vi "Streaming.vi"(9 "Image Display Refnum":refnum<vi>, 10 "OnOff Refnum":refnum<vi>, 11 "camera":u64) -> ()   [LabVIEW 2019]
uses:
  EmergentCameraC/EmergentCameraC.lvlib
panel:
  in  "dshould":i32
  in  "dusing":i32
  in  "frame2":T1
  in  "frame1":T1
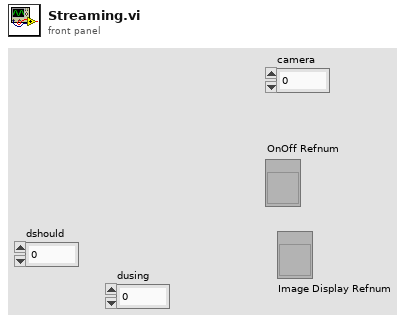
[diagram p1: front panel]
types:
  T1 = cluster{"pixel_type":u32, "size_x":u32, "size_y":u32, "stride":i32, "offset_x":u32, "offset_y":u32, "padding_x":u32, "padding_y":u32, "trailer_size_y":u32, "frame_id":u16, "@dummy control@":i8, "@dummy control@":i8, "imagePtr":i64, "bufferSize":u32, "@dummy control@":i8, "@dummy control@":i8, "@dummy control@":i8, "@dummy control@":i8, "timestamp":u64, "nsecs":u64, "convertColor":i32, "convertBitDepth":i32, "privateData[0]":u8, "privateData[1]":u8, "privateData[2]":u8, "privateData[3]":u8, "privateData[4]":u8, "privateData[5]":u8, "privateData[6]":u8, "privateData[7]":u8, "privateData[8]":u8, "privateData[9]":u8, "privateData[10]":u8, "privateData[11]":u8, "privateData[12]":u8, "privateData[13]":u8, "privateData[14]":u8, "privateData[15]":u8, "privateData[16]":u8, "privateData[17]":u8, "privateData[18]":u8, "privateData[19]":u8, "privateData[20]":u8, "privateData[21]":u8, "privateData[22]":u8, "privateData[23]":u8, "privateData[24]":u8, "privateData[25]":u8, "privateData[26]":u8, "privateData[27]":u8, "privateData[28]":u8, "privateData[29]":u8, "privateData[30]":u8, "privateData[31]":u8, "privateData[32]":u8, "privateData[33]":u8, "privateData[34]":u8, "privateData[35]":u8, "privateData[36]":u8, "privateData[37]":u8, "privateData[38]":u8, "privateData[39]":u8, "privateData[40]":u8, "privateData[41]":u8, "privateData[42]":u8, "privateData[43]":u8, "privateData[44]":u8, "privateData[45]":u8, "privateData[46]":u8, "privateData[47]":u8, "privateData[48]":u8, "privateData[49]":u8, "privateData[50]":u8, "privateData[51]":u8, "privateData[52]":u8, "privateData[53]":u8, "privateData[54]":u8, "privateData[55]":u8, "privateData[56]":u8, "privateData[57]":u8, "privateData[58]":u8, "privateData[59]":u8, "privateData[60]":u8, "privateData[61]":u8, "privateData[62]":u8, "privateData[63]":u8, "privateData[64]":u8, "privateData[65]":u8, "privateData[66]":u8, "privateData[67]":u8, "privateData[68]":u8, "privateData[69]":u8, "privateData[70]":u8, "privateData[71]":u8, "privateData[72]":u8, "privateData[73]":u8, "privateData[74]":u8, "privateData[75]":u8, "privateData[76]":u8, "privateData[77]":u8, "privateData[78]":u8, "privateData[79]":u8, "privateData[80]":u8, "privateData[81]":u8, "privateData[82]":u8, "privateData[83]":u8, "privateData[84]":u8, "privateData[85]":u8, "privateData[86]":u8, "privateData[87]":u8, "privateData[88]":u8, "privateData[89]":u8, "privateData[90]":u8, "privateData[91]":u8, "privateData[92]":u8, "privateData[93]":u8, "privateData[94]":u8, "privateData[95]":u8, "privateData[96]":u8, "privateData[97]":u8, "privateData[98]":u8, "privateData[99]":u8, "privateData[100]":u8, "privateData[101]":u8, "privateData[102]":u8, "privateData[103]":u8, "privateData[104]":u8, "privateData[105]":u8, "privateData[106]":u8, "privateData[107]":u8, "privateData[108]":u8, "privateData[109]":u8, "privateData[110]":u8, "privateData[111]":u8, "privateData[112]":u8, "privateData[113]":u8, "privateData[114]":u8, "privateData[115]":u8, "privateData[116]":u8, "privateData[117]":u8, "privateData[118]":u8, "privateData[119]":u8, "privateData[120]":u8, "privateData[121]":u8, "privateData[122]":u8, "privateData[123]":u8, "privateData[124]":u8, "privateData[125]":u8, "privateData[126]":u8, "privateData[127]":u8, "privateData[128]":u8, "privateData[129]":u8, "privateData[130]":u8, "privateData[131]":u8, "privateData[132]":u8, "privateData[133]":u8, "privateData[134]":u8, "privateData[135]":u8, "privateData[136]":u8, "privateData[137]":u8, "privateData[138]":u8, "privateData[139]":u8, "privateData[140]":u8, "privateData[141]":u8, "privateData[142]":u8, "privateData[143]":u8, "privateData[144]":u8, "privateData[145]":u8, "privateData[146]":u8, "privateData[147]":u8, "privateData[148]":u8, "privateData[149]":u8, "privateData[150]":u8, "privateData[151]":u8, "privateData[152]":u8, "privateData[153]":u8, "privateData[154]":u8, "privateData[155]":u8, "privateData[156]":u8, "privateData[157]":u8, "privateData[158]":u8, "privateData[159]":u8, "privateData[160]":u8, "privateData[161]":u8, "privateData[162]":u8, "privateData[163]":u8, "privateData[164]":u8, "privateData[165]":u8, "privateData[166]":u8, "privateData[167]":u8, "privateData[168]":u8, "privateData[169]":u8, "privateData[170]":u8, "privateData[171]":u8, "privateData[172]":u8, "privateData[173]":u8, "privateData[174]":u8, "privateData[175]":u8, "privateData[176]":u8, "privateData[177]":u8, "privateData[178]":u8, "privateData[179]":u8, "privateData[180]":u8, "privateData[181]":u8, "privateData[182]":u8, "privateData[183]":u8, "privateData[184]":u8, "privateData[185]":u8, "privateData[186]":u8, "privateData[187]":u8, "privateData[188]":u8, "privateData[189]":u8, "privateData[190]":u8, "privateData[191]":u8, "privateData[192]":u8, "privateData[193]":u8, "privateData[194]":u8, "privateData[195]":u8, "privateData[196]":u8, "privateData[197]":u8, "privateData[198]":u8, "privateData[199]":u8, "privateData[200]":u8, "privateData[201]":u8, "privateData[202]":u8, "privateData[203]":u8, "privateData[204]":u8, "privateData[205]":u8, "privateData[206]":u8, "privateData[207]":u8, "privateData[208]":u8, "privateData[209]":u8, "privateData[210]":u8, "privateData[211]":u8, "privateData[212]":u8, "privateData[213]":u8, "privateData[214]":u8, "privateData[215]":u8, "privateData[216]":u8, "privateData[217]":u8, "privateData[218]":u8, "privateData[219]":u8, "privateData[220]":u8, "privateData[221]":u8, "privateData[222]":u8, "privateData[223]":u8, "privateData[224]":u8, "privateData[225]":u8, "privateData[226]":u8, "privateData[227]":u8, "privateData[228]":u8, "privateData[229]":u8, "privateData[230]":u8, "privateData[231]":u8, "privateData[232]":u8, "privateData[233]":u8, "privateData[234]":u8, "privateData[235]":u8, "privateData[236]":u8, "privateData[237]":u8, "privateData[238]":u8, "privateData[239]":u8, "privateData[240]":u8, "privateData[241]":u8, "privateData[242]":u8, "privateData[243]":u8, "privateData[244]":u8, "privateData[245]":u8, "privateData[246]":u8, "privateData[247]":u8, "privateData[248]":u8, "privateData[249]":u8, "privateData[250]":u8, "privateData[251]":u8, "privateData[252]":u8, "privateData[253]":u8, "privateData[254]":u8, "privateData[255]":u8}
  T2 = cluster{"pixel_type":u32, "size_x":u32, "size_y":u32, "stride":i32, "offset_x":u32, "offset_y":u32, "padding_x":u32, "padding_y":u32, "trailer_size_y":u32, "frame_id":u16, "@dummy control@":i8, "@dummy control@":i8, "imagePtr":i64, "bufferSize":u32, "@dummy control@":i8, "@dummy control@":i8, "@dummy control@":i8, "@dummy control@":i8, "timestamp":u64, "nsecs":u64, "convertColor":i32, "convertBitDepth":i32, "privateData[0]":u8, "privateData[1]":u8, "privateData[2]":u8, "privateData[3]":u8, "privateData[4]":u8, "privateData[5]":u8, "privateData[6]":u8, "privateData[7]":u8, "privateData[8]":u8, "privateData[9]":u8, "privateData[10]":u8, "privateData[11]":u8, "privateData[12]":u8, "privateData[13]":u8, "privateData[14]":u8, "privateData[15]":u8, "privateData[16]":u8, "privateData[17]":u8, "privateData[18]":u8, "privateData[19]":u8, "privateData[20]":u8, "privateData[21]":u8, "privateData[22]":u8, "privateData[23]":u8, "privateData[24]":u8, "privateData[25]":u8, "privateData[26]":u8, "privateData[27]":u8, "privateData[28]":u8, "privateData[29]":u8, "privateData[30]":u8, "privateData[31]":u8, "privateData[32]":u8, "privateData[33]":u8, "privateData[34]":u8, "privateData[35]":u8, "privateData[36]":u8, "privateData[37]":u8, "privateData[38]":u8, "privateData[39]":u8, "privateData[40]":u8, "privateData[41]":u8, "privateData[42]":u8, "privateData[43]":u8, "privateData[44]":u8, "privateData[45]":u8, "privateData[46]":u8, "privateData[47]":u8, "privateData[48]":u8, "privateData[49]":u8, "privateData[50]":u8, "privateData[51]":u8, "privateData[52]":u8, "privateData[53]":u8, "privateData[54]":u8, "privateData[55]":u8, "privateData[56]":u8, "privateData[57]":u8, "privateData[58]":u8, "privateData[59]":u8, "privateData[60]":u8, "privateData[61]":u8, "privateData[62]":u8, "privateData[63]":u8, "privateData[64]":u8, "privateData[65]":u8, "privateData[66]":u8, "privateData[67]":u8, "privateData[68]":u8, "privateData[69]":u8, "privateData[70]":u8, "privateData[71]":u8, "privateData[72]":u8, "privateData[73]":u8, "privateData[74]":u8, "privateData[75]":u8, "privateData[76]":u8, "privateData[77]":u8, "privateData[78]":u8, "privateData[79]":u8, "privateData[80]":u8, "privateData[81]":u8, "privateData[82]":u8, "privateData[83]":u8, "privateData[84]":u8, "privateData[85]":u8, "privateData[86]":u8, "privateData[87]":u8, "privateData[88]":u8, "privateData[89]":u8, "privateData[90]":u8, "privateData[91]":u8, "privateData[92]":u8, "privateData[93]":u8, "privateData[94]":u8, "privateData[95]":u8, "privateData[96]":u8, "privateData[97]":u8, "privateData[98]":u8, "privateData[99]":u8, "privateData[100]":u8, "privateData[101]":u8, "privateData[102]":u8, "privateData[103]":u8, "privateData[104]":u8, "privateData[105]":u8, "privateData[106]":u8, "privateData[107]":u8, "privateData[108]":u8, "privateData[109]":u8, "privateData[110]":u8, "privateData[111]":u8, "privateData[112]":u8, "privateData[113]":u8, "privateData[114]":u8, "privateData[115]":u8, "privateData[116]":u8, "privateData[117]":u8, "privateData[118]":u8, "privateData[119]":u8, "privateData[120]":u8, "privateData[121]":u8, "privateData[122]":u8, "privateData[123]":u8, "privateData[124]":u8, "privateData[125]":u8, "privateData[126]":u8, "privateData[127]":u8, "privateData[128]":u8, "privateData[129]":u8, "privateData[130]":u8, "privateData[131]":u8, "privateData[132]":u8, "privateData[133]":u8, "privateData[134]":u8, "privateData[135]":u8, "privateData[136]":u8, "privateData[137]":u8, "privateData[138]":u8, "privateData[139]":u8, "privateData[140]":u8, "privateData[141]":u8, "privateData[142]":u8, "privateData[143]":u8, "privateData[144]":u8, "privateData[145]":u8, "privateData[146]":u8, "privateData[147]":u8, "privateData[148]":u8, "privateData[149]":u8, "privateData[150]":u8, "privateData[151]":u8, "privateData[152]":u8, "privateData[153]":u8, "privateData[154]":u8, "privateData[155]":u8, "privateData[156]":u8, "privateData[157]":u8, "privateData[158]":u8, "privateData[159]":u8, "privateData[160]":u8, "privateData[161]":u8, "privateData[162]":u8, "privateData[163]":u8, "privateData[164]":u8, "privateData[165]":u8, "privateData[166]":u8, "privateData[167]":u8, "privateData[168]":u8, "privateData[169]":u8, "privateData[170]":u8, "privateData[171]":u8, "privateData[172]":u8, "privateData[173]":u8, "privateData[174]":u8, "privateData[175]":u8, "privateData[176]":u8, "privateData[177]":u8, "privateData[178]":u8, "privateData[179]":u8, "privateData[180]":u8, "privateData[181]":u8, "privateData[182]":u8, "privateData[183]":u8, "privateData[184]":u8, "privateData[185]":u8, "privateData[186]":u8, "privateData[187]":u8, "privateData[188]":u8, "privateData[189]":u8, "privateData[190]":u8, "privateData[191]":u8, "privateData[192]":u8, "privateData[193]":u8, "privateData[194]":u8, "privateData[195]":u8, "privateData[196]":u8, "privateData[197]":u8, "privateData[198]":u8, "privateData[199]":u8, "privateData[200]":u8, "privateData[201]":u8, "privateData[202]":u8, "privateData[203]":u8, "privateData[204]":u8, "privateData[205]":u8, "privateData[206]":u8, "privateData[207]":u8, "privateData[208]":u8, "privateData[209]":u8, "privateData[210]":u8, "privateData[211]":u8, "privateData[212]":u8, "privateData[213]":u8, "privateData[214]":u8, "privateData[215]":u8, "privateData[216]":u8, "privateData[217]":u8, "privateData[218]":u8, "privateData[219]":u8, "privateData[220]":u8, "privateData[221]":u8, "privateData[222]":u8, "privateData[223]":u8, "privateData[224]":u8, "privateData[225]":u8, "privateData[226]":u8, "privateData[227]":u8, "privateData[228]":u8, "privateData[229]":u8, "privateData[230]":u8, "privateData[231]":u8, "privateData[232]":u8, "privateData[233]":u8, "privateData[234]":u8, "privateData[235]":u8, "privateData[236]":u8, "privateData[237]":u8, "privateData[238]":u8, "privateData[239]":u8, "privateData[240]":u8, "privateData[241]":u8, "privateData[242]":u8, "privateData[243]":u8, "privateData[244]":u8, "privateData[245]":u8, "privateData[246]":u8, "privateData[247]":u8, "privateData[248]":u8, "privateData[249]":u8, "privateData[250]":u8, "privateData[251]":u8, "privateData[252]":u8, "privateData[253]":u8, "privateData[254]":u8, "privateData[255]":u8}[]
  T3 = typedef "Image Type" = u32
  T4 = typedef "Semaphore RefNum" = refnum<k1>
  T5 = typedef "IMAQ Image.ctl" = refnum<image>
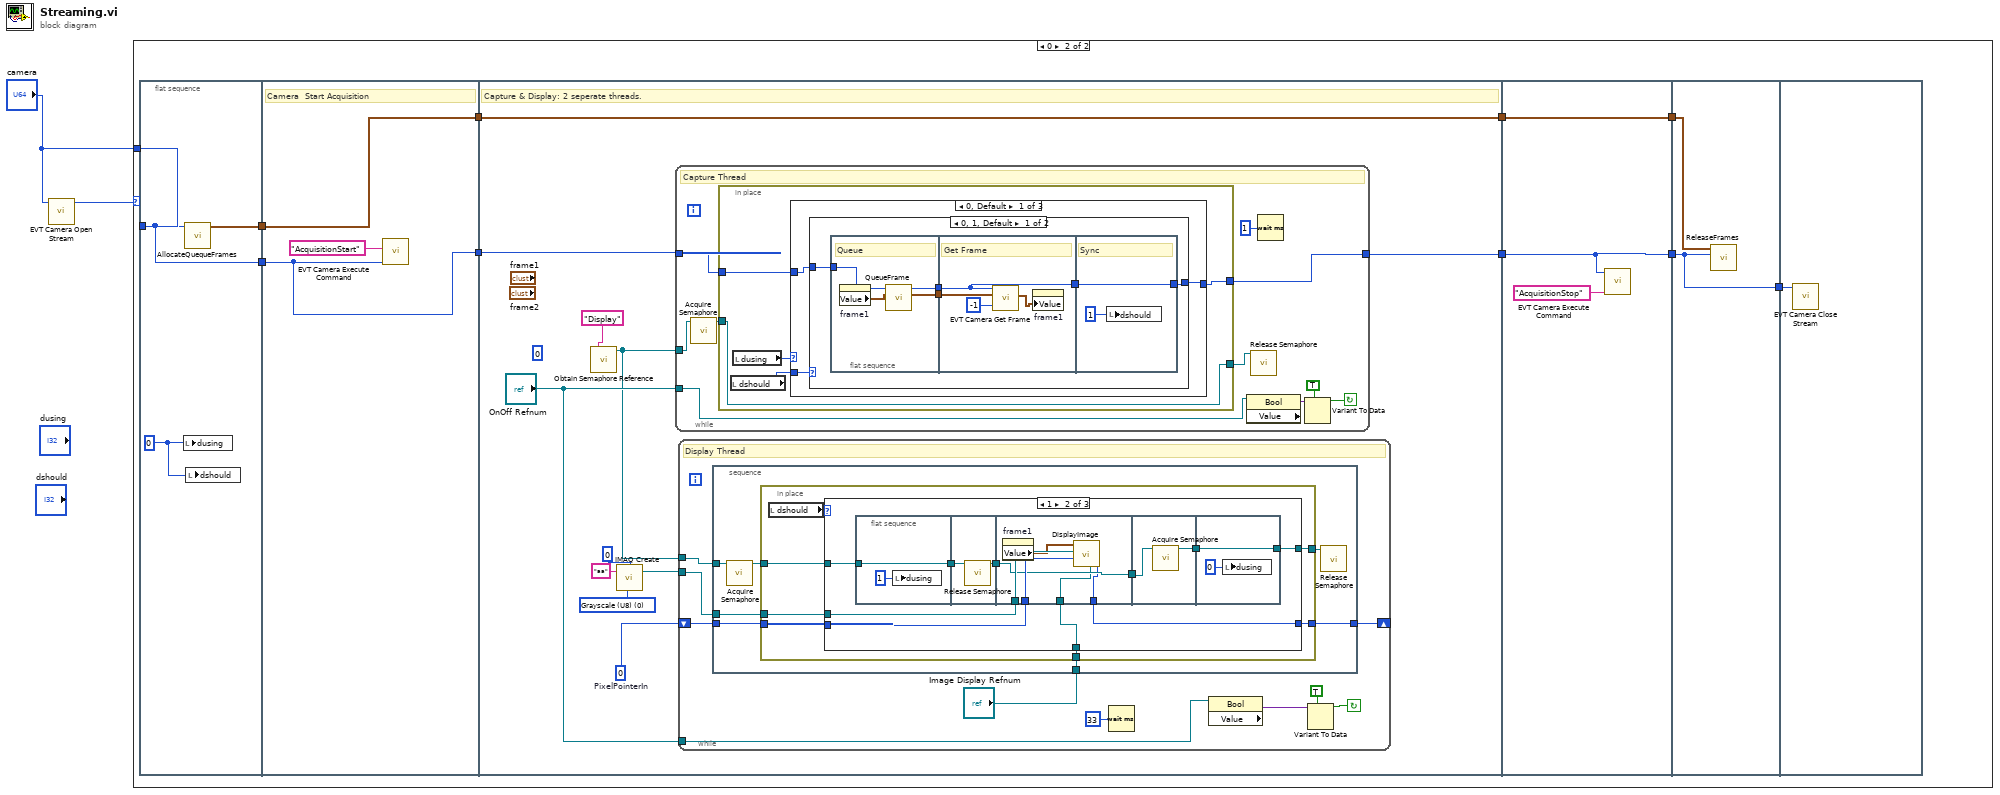
[diagram p0: block diagram]
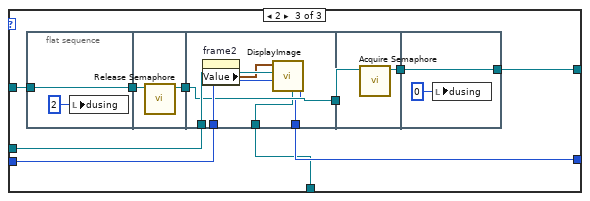
[diagram p4: hidden frame]
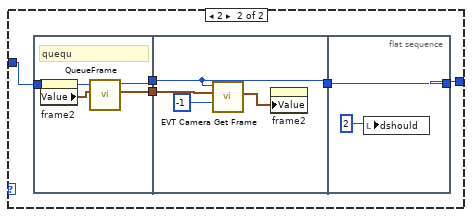
[diagram p5: hidden frame]
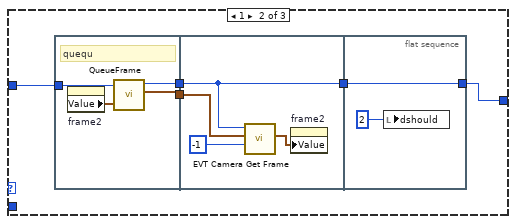
[diagram p6: hidden frame]
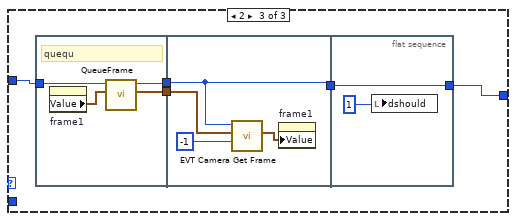
[diagram p7: hidden frame]
diagram:
  n1 = call "EVT Camera Open Stream.vi"("camera"="camera") -> ("function return"=w1:u32)  [unwired: 10 in]
  n2 = case shown="0" w1 {
    tunnel: "camera" -> [_ w3]
    frame Default {
    }
    frame 0 {
      n3 = flat-sequence {
        tunnel: [w15] -> w12
        tunnel: w3 -> [w14]
        tunnel: [w14] -> w11
        tunnel: w12 -> [w18]
        tunnel: w11 -> [w17]
        tunnel: [w18] -> w10
        tunnel: [w17] -> w4
        tunnel: w10 -> [w29]
        tunnel: [w28] -> w9
        tunnel: [w29] -> w8
        tunnel: w4 -> [w27]
        tunnel: w9 -> [w183]
        tunnel: w8 -> [w182]
        tunnel: [w183] -> w7
        tunnel: [w182] -> w6
        tunnel: w7 -> [w185]
        tunnel: w6 -> [w186]
        tunnel: [w185] -> w5
        tunnel: w5 -> [w187]
        frame #0 {
          w13 = 0 ("frameDisplayUse")
          n4 = local write "dusing"(w13) -> ()
          n5 = call "AllocateQuequeFrames.vi"("camera"=w14) -> ("Array"=w15:T2)  [unwired: 9 in, 1 out]
          n6 = local write "dshould"(w13) -> ()
        }
        frame #1 {
          # "Camera  Start Acquisition"
          n7 = call "EVT Camera Execute Command.vi"("name"="AcquisitionStart", "camera"=w17) -> ()  [unwired: 9 in, 1 out]
        }
        frame #2 {
          w19 = T3 0 items=["Grayscale (U8)", "Grayscale (I16)", "Grayscale (SGL)", "Complex (CSG)", "RGB (U32)", "HSL (U32)", "RGB (U64)", "Grayscale (U16)"] ("Image Type")
          w21 = u64 0  # PixelPointerIn
          (unwired) u16 0 ("op")
          # "Capture & Display: 2 seperate threads."
          n8 = call <vilib>:"Obtain Semaphore Reference.vi"("name (unnamed)"="Display") -> ("semaphore"=w24:T4)  [unwired: 4 in, 2 out]
          n9 = call "IMAQ Create"("Border Size"=0, "Image Name"="aa", "Image Type"=w19) -> ("New Image"=w20:T5)  [unwired: 2 in, 1 out]
          n10 = while "Capture thread" {
            tunnel: w27 -> [w108]
            tunnel: [w104] -> w28
            tunnel: w24 -> [w109]
            tunnel: "OnOff Refnum" -> [w105]
            stop <- w110 continue-if-true
            # "Capture Thread"
            n11 = call <vilib>:"Acquire Semaphore.vi"("semaphore"=w109) -> ("semaphore out"=w107:T4)  [unwired: 4 in, 2 out]
            n12 = in-place {
              in-place-border: w108 -> [w118]
              in-place-border: w107 -> [w115]
              in-place-border: [w115] -> w106
              in-place-border: [w114] -> w104
              n13 = local read "dshould"() -> (w116:i32)
              n14 = local read "dusing"() -> (w117:i32)
              n15 = case shown="0, Default" w117 {
                tunnel: w118 -> [w121 w154 w168]
                tunnel: [w120 w152 w167] -> w114
                tunnel: w116 -> [w119 _ _]
                frame 0, Default {
                  n16 = case shown="0, 1, Default" w119 {
                    tunnel: w121 -> [w124 w137]
                    tunnel: [w123 w138] -> w120
                    frame 0, 1, Default {
                      n17 = flat-sequence {
                        tunnel: w124 -> [w130]
                        tunnel: [w127] -> w126
                        tunnel: [w129] -> w122
                        tunnel: w126 -> [w133]
                        tunnel: [w132] -> w125
                        tunnel: w122 -> [w132]
                        tunnel: [w136] -> w123
                        tunnel: w125 -> [w136]
                        frame #0 {
                          # "Queue"
                          n18 = property on="frame1" class="Clust (strict)"() -> ("Value"=w128:T1)  [unwired: 2 in, 2 out]
                          n19 = call "QueueFrame.vi"("frame"=w128, "camera"=w130) -> ("frame_out"=w127:T1, "camera_out"=w129:u64)  [unwired: 8 in]
                        }
                        frame #1 {
                          # "Get Frame"
                          n20 = call "EVT Camera Get Frame.vi"("timeout"=-1, "frame"=w133, "camera"=w132) -> ("frame out"=w131:T1)  [unwired: 7 in, 1 out]
                          n21 = property on="frame1" class="Clust (strict)"("Value"=w131) -> ()  [unwired: 2 in, 2 out]
                        }
                        frame #2 {
                          # "Sync"
                          n22 = local write "dshould"(1 ("DisplayFrame")) -> ()
                        }
                      }
                    }
                    frame 2 {
                      n23 = flat-sequence {
                        tunnel: w137 -> [w145]
                        tunnel: [w143] -> w141
                        tunnel: [w144] -> w140
                        tunnel: w141 -> [w148]
                        tunnel: w140 -> [w147]
                        tunnel: [w147] -> w139
                        tunnel: [w150] -> w138
                        tunnel: w139 -> [w150]
                        frame #0 {
                          # "quequ"
                          n24 = property on="frame2" class="Clust (strict)"() -> ("Value"=w142:T1)  [unwired: 2 in, 2 out]
                          n25 = call "QueueFrame.vi"("frame"=w142, "camera"=w145) -> ("frame_out"=w143:T1, "camera_out"=w144:u64)  [unwired: 8 in]
                        }
                        frame #1 {
                          n26 = call "EVT Camera Get Frame.vi"("timeout"=-1, "frame"=w148, "camera"=w147) -> ("frame out"=w146:T1)  [unwired: 7 in, 1 out]
                          n27 = property on="frame2" class="Clust (strict)"("Value"=w146) -> ()  [unwired: 2 in, 2 out]
                        }
                        frame #2 {
                          n28 = local write "dshould"(2 ("DisplayFrame")) -> ()
                        }
                      }
                    }
                  }
                }
                frame 1 {
                  n29 = flat-sequence {
                    tunnel: w154 -> [w160]
                    tunnel: [w158] -> w156
                    tunnel: [w159] -> w155
                    tunnel: w156 -> [w163]
                    tunnel: w155 -> [w162]
                    tunnel: [w162] -> w153
                    tunnel: [w165] -> w152
                    tunnel: w153 -> [w165]
                    frame #0 {
                      # "quequ"
                      n30 = property on="frame2" class="Clust (strict)"() -> ("Value"=w157:T1)  [unwired: 2 in, 2 out]
                      n31 = call "QueueFrame.vi"("frame"=w157, "camera"=w160) -> ("frame_out"=w158:T1, "camera_out"=w159:u64)  [unwired: 8 in]
                    }
                    frame #1 {
                      n32 = call "EVT Camera Get Frame.vi"("timeout"=-1, "frame"=w163, "camera"=w162) -> ("frame out"=w161:T1)  [unwired: 7 in, 1 out]
                      n33 = property on="frame2" class="Clust (strict)"("Value"=w161) -> ()  [unwired: 2 in, 2 out]
                    }
                    frame #2 {
                      n34 = local write "dshould"(2 ("DisplayFrame")) -> ()
                    }
                  }
                }
                frame 2 {
                  n35 = flat-sequence {
                    tunnel: w168 -> [w175]
                    tunnel: [w173] -> w171
                    tunnel: [w174] -> w170
                    tunnel: w171 -> [w178]
                    tunnel: w170 -> [w177]
                    tunnel: [w177] -> w169
                    tunnel: [w181] -> w167
                    tunnel: w169 -> [w181]
                    frame #0 {
                      # "quequ"
                      n36 = property on="frame1" class="Clust (strict)"() -> ("Value"=w172:T1)  [unwired: 2 in, 2 out]
                      n37 = call "QueueFrame.vi"("frame"=w172, "camera"=w175) -> ("frame_out"=w173:T1, "camera_out"=w174:u64)  [unwired: 8 in]
                    }
                    frame #1 {
                      n38 = call "EVT Camera Get Frame.vi"("timeout"=-1, "frame"=w178, "camera"=w177) -> ("frame out"=w176:T1)  [unwired: 7 in, 1 out]
                      n39 = property on="frame1" class="Clust (strict)"("Value"=w176) -> ()  [unwired: 2 in, 2 out]
                    }
                    frame #2 {
                      n40 = local write "dshould"(1 ("DisplayFrame")) -> ()
                    }
                  }
                }
              }
            }
            n41 = property class="Bool"(reference=w105) -> ("Value"=w112:variant)  [unwired: 1 in, 2 out]
            n42 = call <vilib>:"Release Semaphore.vi"("semaphore"=w106) -> ()  [unwired: 5 in, 2 out]
            n43 = Wait (ms)(milliseconds to wait=u32 1) -> ()  [unwired: 1 out]
            n44 = Variant To Data(type=TRUE, Variant=w112) -> (data=w110:bool)  [unwired: 1 in, 1 out]
          }
          n45 = while {
            tunnel: w20 -> [w33]
            shift-right: [w32] -> _
            shift-left: w21 -> [w34]
            tunnel: w24 -> [w35]
            tunnel: "OnOff Refnum" -> [w30]
            stop <- w36 continue-if-true
            # "Display Thread"
            n46 = stacked-sequence {
              tunnel: w34 -> [w46]
              tunnel: w35 -> [w45]
              tunnel: w33 -> [w43]
              tunnel: [w42] -> w32
              tunnel: "Image Display Refnum" -> [w40]
              frame #0 {
                n47 = call <vilib>:"Acquire Semaphore.vi"("semaphore"=w45) -> ("semaphore out"=w44:T4)  [unwired: 4 in, 2 out]
                n48 = in-place {
                  in-place-border: w46 -> [w52]
                  in-place-border: w44 -> [w51]
                  in-place-border: w43 -> [w50]
                  in-place-border: [w49] -> w41
                  in-place-border: [w48] -> w42
                  in-place-border: w40 -> [w47]
                  n49 = local read "dshould"() -> (w53:i32)
                  n50 = case shown="1" w53 {
                    tunnel: w52 -> [w54 w62 w86]
                    tunnel: w51 -> [w55 w65 w89]
                    tunnel: w50 -> [_ w63 w87]
                    tunnel: [w55 w58 w82] -> w49
                    tunnel: [w54 w57 w81] -> w48
                    tunnel: w47 -> [_ w56 w80]
                    frame 0, Default {
                    }
                    frame 1 {
                      n51 = flat-sequence {
                        tunnel: w65 -> [w66]
                        tunnel: [w66] -> w64
                        tunnel: w64 -> [w69]
                        tunnel: [w68] -> w61
                        tunnel: w63 -> [w75]
                        tunnel: w62 -> [w74]
                        tunnel: w61 -> [w73]
                        tunnel: [w73] -> w60
                        tunnel: [w72] -> w57
                        tunnel: w56 -> [w71]
                        tunnel: w60 -> [w77]
                        tunnel: [w76] -> w59
                        tunnel: [w79] -> w58
                        tunnel: w59 -> [w79]
                        frame #0 {
                          n52 = local write "dusing"(1 ("dusing")) -> ()
                        }
                        frame #1 {
                          n53 = call <vilib>:"Release Semaphore.vi"("semaphore"=w69) -> ("semaphore out"=w68:T4)  [unwired: 5 in, 1 out]
                        }
                        frame #2 {
                          n54 = property on="frame1" class="Clust (strict)"() -> ("Value"=w70:T1)  [unwired: 2 in, 2 out]
                          n55 = call "DisplayImage.vi"("frame"=w70, "ImageIMAQ"=w75, "PixelPointerIn"=w74, "Image Display Refnum"=w71) -> ("PixelPointerOut"=w72:u64)  [unwired: 4 in, 1 out]
                        }
                        frame #3 {
                          n56 = call <vilib>:"Acquire Semaphore.vi"("semaphore"=w77) -> ("semaphore out"=w76:T4)  [unwired: 4 in, 2 out]
                        }
                        frame #4 {
                          n57 = local write "dusing"(0 ("dusing")) -> ()
                        }
                      }
                    }
                    frame 2 {
                      n58 = flat-sequence {
                        tunnel: w89 -> [w90]
                        tunnel: [w90] -> w88
                        tunnel: w88 -> [w93]
                        tunnel: [w92] -> w85
                        tunnel: w87 -> [w99]
                        tunnel: w86 -> [w98]
                        tunnel: w85 -> [w97]
                        tunnel: [w97] -> w84
                        tunnel: [w96] -> w81
                        tunnel: w80 -> [w95]
                        tunnel: w84 -> [w101]
                        tunnel: [w100] -> w83
                        tunnel: [w103] -> w82
                        tunnel: w83 -> [w103]
                        frame #0 {
                          n59 = local write "dusing"(2 ("dusing")) -> ()
                        }
                        frame #1 {
                          n60 = call <vilib>:"Release Semaphore.vi"("semaphore"=w93) -> ("semaphore out"=w92:T4)  [unwired: 5 in, 1 out]
                        }
                        frame #2 {
                          n61 = property on="frame2" class="Clust (strict)"() -> ("Value"=w94:T1)  [unwired: 2 in, 2 out]
                          n62 = call "DisplayImage.vi"("frame"=w94, "ImageIMAQ"=w99, "PixelPointerIn"=w98, "Image Display Refnum"=w95) -> ("PixelPointerOut"=w96:u64)  [unwired: 4 in, 1 out]
                        }
                        frame #3 {
                          n63 = call <vilib>:"Acquire Semaphore.vi"("semaphore"=w101) -> ("semaphore out"=w100:T4)  [unwired: 4 in, 2 out]
                        }
                        frame #4 {
                          n64 = local write "dusing"(0 ("dusing")) -> ()
                        }
                      }
                    }
                  }
                }
                n65 = call <vilib>:"Release Semaphore.vi"("semaphore"=w41) -> ()  [unwired: 5 in, 2 out]
              }
            }
            n66 = Wait (ms)(milliseconds to wait=u32 33) -> ()  [unwired: 1 out]
            n67 = property class="Bool"(reference=w30) -> ("Value"=w38:variant)  [unwired: 1 in, 2 out]
            n68 = Variant To Data(type=TRUE, Variant=w38) -> (data=w36:bool)  [unwired: 1 in, 1 out]
          }
        }
        frame #3 {
          n69 = call "EVT Camera Execute Command.vi"("name"="AcquisitionStop", "camera"=w183) -> ()  [unwired: 9 in, 1 out]
        }
        frame #4 {
          n70 = call "ReleaseFrames.vi"("camera"=w185, "Array"=w186) -> ()  [unwired: 10 in]
        }
        frame #5 {
          n71 = call "EVT Camera Close Stream.vi"("camera"=w187) -> ()  [unwired: 10 in, 1 out]
        }
      }
    }
  }
